vi "UMB_GTFO.vi"(11 "IR distance":dbl) -> (3 "Behavior Output":T1)   [LabVIEW 2012]
uses:
  NINJA Code/Tugboat/Robo_Programs/behaviorOutput_t.ctl
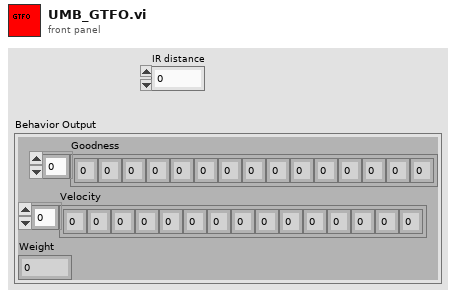
[diagram p1: front panel]
types:
  T1 = typedef "behaviorOutput_t.ctl" = cluster{"Goodness":i8[], "Velocity":i8[], "Weight":i8}
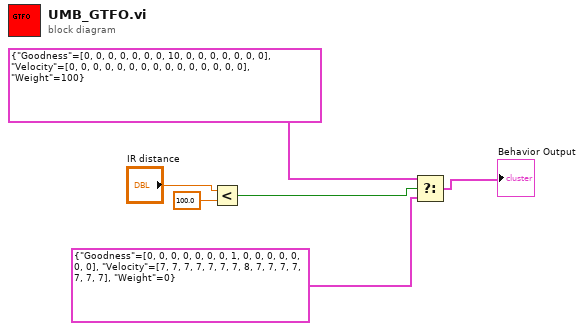
[diagram p0: block diagram]
diagram:
  n1 = Less?(x="IR distance", y=100.0) -> (x < y?=w1:bool)
  n2 = Select(t=T1 {"Goodness"=[0, 0, 0, 0, 0, 0, 0, 10, 0, 0, 0, 0, 0, 0, 0], "Velocity"=[0, 0, 0, 0, 0, 0, 0, 0, 0, 0, 0, 0, 0, 0, 0], "Weight"=100} ("Behavior Output"), s=w1, f=T1 {"Goodness"=[0, 0, 0, 0, 0, 0, 0, 1, 0, 0, 0, 0, 0, 0, 0], "Velocity"=[7, 7, 7, 7, 7, 7, 7, 8, 7, 7, 7, 7, 7, 7, 7], "Weight"=0} ("Behavior Output")) -> (s? t:f=→"Behavior Output":T1)
